vi "Generate One Point On Waveform Chart.vi"(1 "Index":i32) -> (0 "waveform chart":cluster{dbl, i32}(graph)={0.5489327770964688, 0})   [LabVIEW 2012]
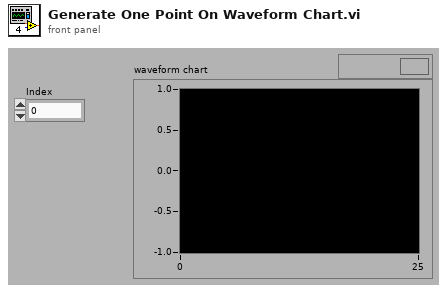
[diagram p1: front panel]
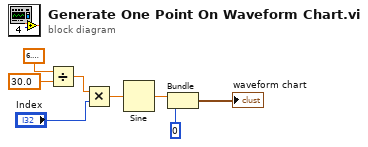
[diagram p0: block diagram]
diagram:
  n1 = Divide(x=6.283185307179586, y=30.0) -> (x/y=w3:dbl)
  n2 = Multiply(x=w3, y="Index") -> (x*y=w5:dbl)
  n3 = Sine(x=w5) -> (sin(x)=w1:dbl)
  n4 = Bundle(w1, 0) -> (→"waveform chart":cluster{dbl, i32})  [unwired: 1 out]
